vi "Measure.vi"(11 "FFmeter settings":T1={"AC Source"={"AC Source type"=enum."Fluke 5XXX calibrator", "VISA"="", "Ref. clock (Hz)"=0.0, "status ref"=refnum}, "TWM pipe"="\\\\.\\pipe\\TWM:server", "Measurement status ref"=refnum, "TWM Status ref"=refnum, "Abort ref"=refnum, "DC meter"={"DC meter type"=enum."H/A/K 3458", "DC meter VISA"="", "NPLC"=10, "No of readings"=3, "status ref"=refnum}, "Measurement properties"={"Measurement frequencies (Hz)"=[1000.0], "Sampling frequency (Hz)"=500000.0, "Signal amplitude (V)"=4.5, "AC-DC settle time (s)"=20.0, "Record length (multiples of period)"=[1000.0, 10000.0, 1000.0], "Measurement template file"=path "", "Row of START keyword"=1, "Row of STOP keyword"=0, "Calculate RMS from samples"=FALSE}} {"Measurement properties"."Record length (multiples of period)" format="%#_3p"; "Measurement properties"."Sampling frequency (Hz)" format="%#_3p"; "Measurement properties"."Measurement frequencies (Hz)" format="%#_3p"}) -> (0 "error out":errorcluster, 3 "FFmeter settings out":T1={"AC Source"={"AC Source type"=enum."Fluke 5XXX calibrator", "VISA"="", "Ref. clock (Hz)"=0.0, "status ref"=refnum}, "TWM pipe"="\\\\.\\pipe\\TWM:server", "Measurement status ref"=refnum, "TWM Status ref"=refnum, "Abort ref"=refnum, "DC meter"={"DC meter type"=enum."H/A/K 3458", "DC meter VISA"="", "NPLC"=10, "No of readings"=3, "status ref"=refnum}, "Measurement properties"={"Measurement frequencies (Hz)"=[1000.0], "Sampling frequency (Hz)"=500000.0, "Signal amplitude (V)"=4.5, "AC-DC settle time (s)"=20.0, "Record length (multiples of period)"=[1000.0, 10000.0, 1000.0], "Measurement template file"=path "", "Row of START keyword"=1, "Row of STOP keyword"=0, "Calculate RMS from samples"=FALSE}} {"Measurement properties"."Record length (multiples of period)" format="%#_3p"; "Measurement properties"."Sampling frequency (Hz)" format="%#_3p"; "Measurement properties"."Measurement frequencies (Hz)" format="%#_3p"})   [LabVIEW 2020]
uses:
  GUI/Type definitions/FFmeter settings.ctl
  General AC source/Type definitions/AC Source.ctl
  General AC source/Type definitions/AC Source type.ctl
  General DC meter/Type definitions/DC meter.ctl
  General DC meter/Type definitions/DC meter type.ctl
  Type definitions/Measuement properties.ctl
  <vilib>/Utility/error.llb/DialogType.ctl
  <vilib>/Utility/NIReport.llb/NI_report.lvclass
  external libraries/varilib/varilib.lvlib
  external libraries/TWM-1.8.7.0-client/TWM Client.lvlib
panel:
  out "offset after":dbl[](array[numeric])
  out "DC readings of AC-AC sequence":dbl[][](array[numeric])
  out "offset before":dbl[](array[numeric])
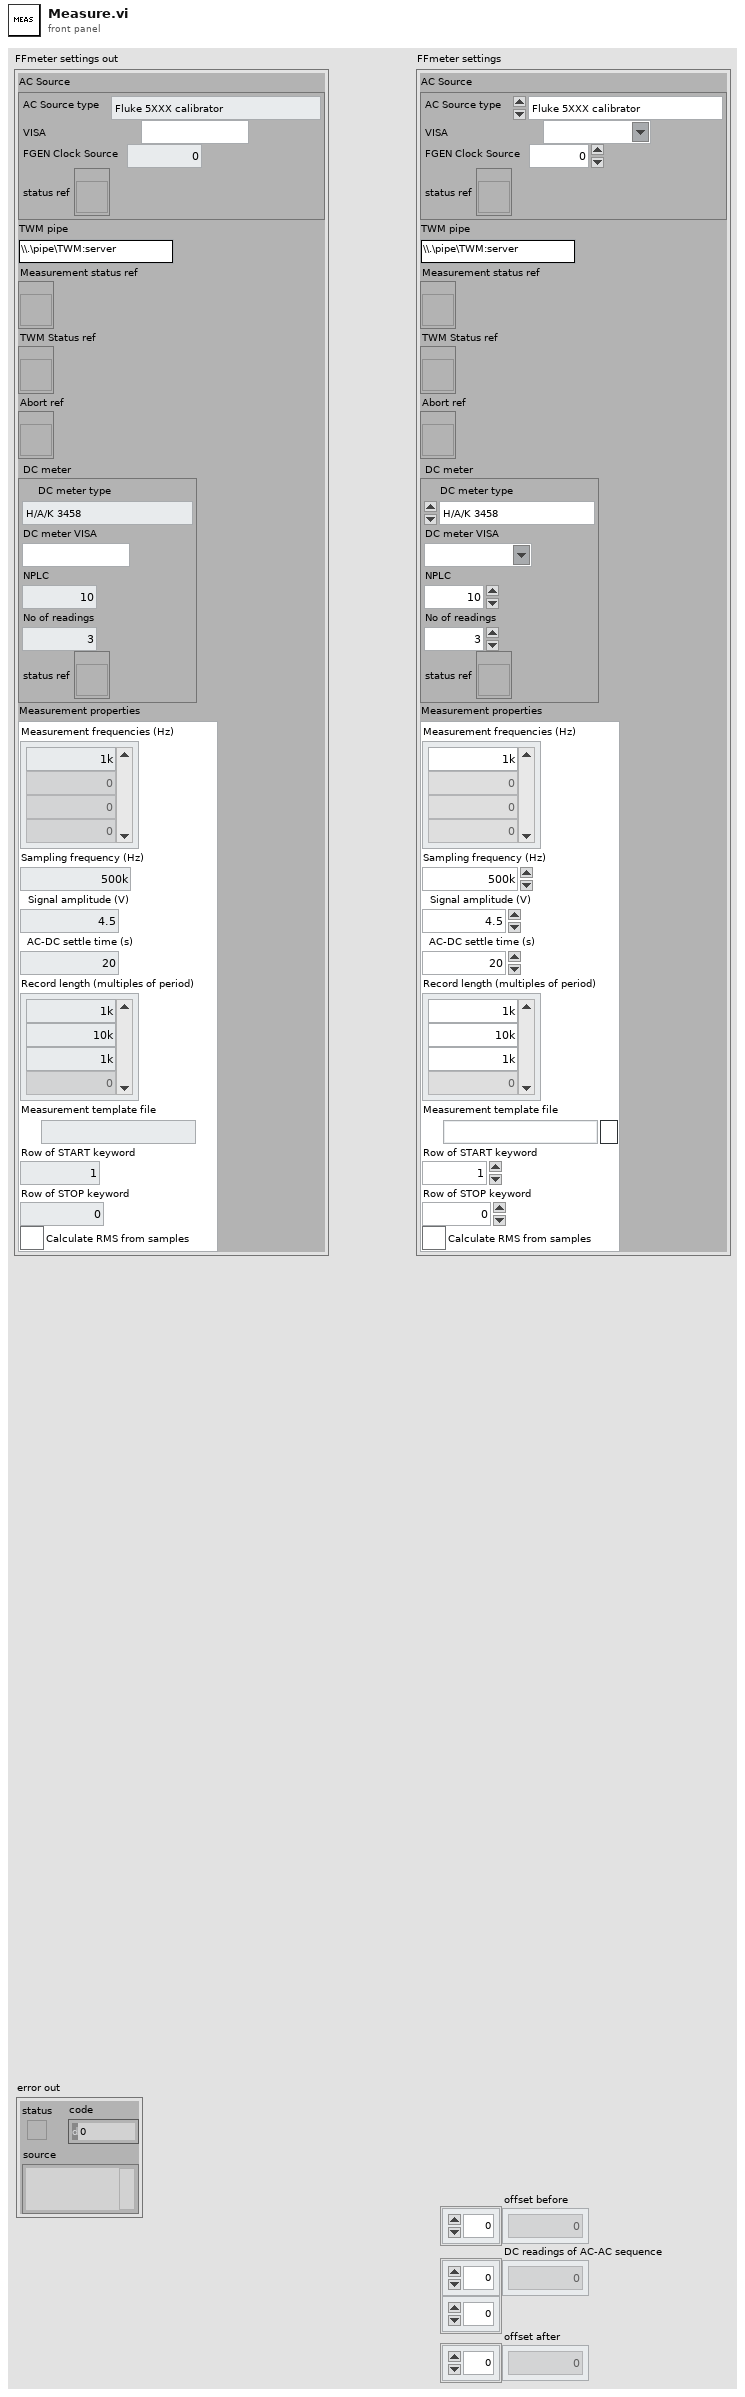
[diagram p1: front panel]
types:
  T1 = typedef "FFmeter settings.ctl" = cluster{"AC Source":T2, "TWM pipe":string, "Measurement status ref":refnum<vi>, "TWM Status ref":refnum<vi>, "Abort ref":refnum<vi>, "DC meter":T4, "Measurement properties":T6}
  T2 = typedef "AC Source.ctl" = cluster{"AC Source type":T3, "VISA":refnum<visa-resource-name>, "Ref. clock (Hz)":dbl, "status ref":refnum<vi>}
  T3 = typedef "AC Source type.ctl" = enum16{"Fluke 5XXX calibrator", "Tektronix AFG3101C", "dummy"}
  T4 = typedef "DC meter.ctl" = cluster{"DC meter type":T5, "DC meter VISA":refnum<visa-resource-name>, "NPLC":i32, "No of readings":i32, "status ref":refnum<vi>}
  T5 = typedef "DC meter type.ctl" = enum16{"H/A/K 3458", "FLuke 8508A", "dummy"}
  T6 = typedef "Measuement properties.ctl" = cluster{"Measurement frequencies (Hz)":dbl[], "Sampling frequency (Hz)":dbl, "Signal amplitude (V)":dbl, "AC-DC settle time (s)":dbl, "Record length (multiples of period)":dbl[], "Measurement template file":path, "Row of START keyword":i32, "Row of STOP keyword":i32, "Calculate RMS from samples":bool}
  T7 = typedef "DialogType.ctl" = u16
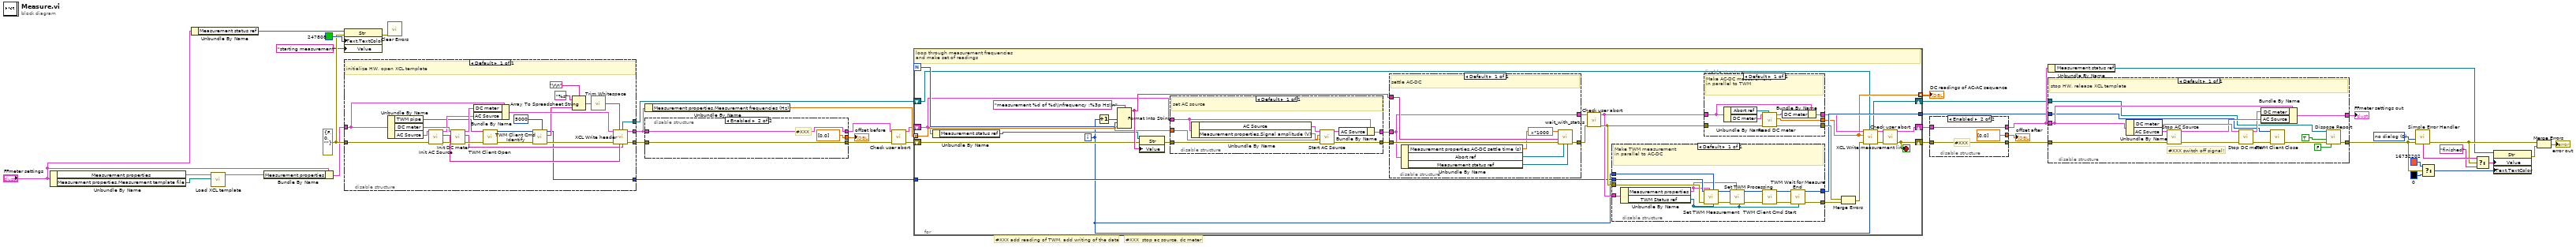
[diagram p0: block diagram]
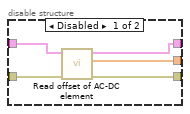
[diagram p2: hidden frame]
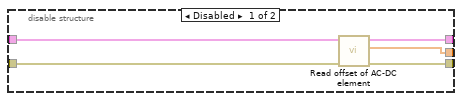
[diagram p3: hidden frame]
diagram:
  w32 = T7 0 items=["no dialog", "OK message", "continue or stop message", "OK message + warnings", "continue/stop + warnings"] ("type of dialog (OK msg:1)")
  w7 = errorcluster {"status"=FALSE, "code"=0, "source"=""} ("error out")
  # "#XXX  stop ac source, dc meter"
  # "#XXX add reading of TWM, add writing of the data"
  n1 = Unbundle By Name("FFmeter settings") -> ("Measurement properties"=w5:T6, "Measurement properties.Measurement template file"=w1:path)
  n2 = Unbundle By Name("FFmeter settings") -> ("Measurement status ref"=w24:refnum<vi>)
  n3 = call "Load XCL template.vi"("Measurement template file"=w1, "Measurement properties"=w5) -> ("Measurement properties out"=w4:T6)  [unwired: 9 in]
  n4 = Bundle By Name(cluster="FFmeter settings", "Measurement properties"=w4) -> (w2:T1)
  n5 = property class="Str"(reference=w24, error in=w7, "Text.TextColor"=u32 247808 ("Text.Text Colors:Text Color"), "Value"="starting measurement") -> (error out=w23:errorcluster)  [unwired: 1 out]
  n6 = disable-structure shown="Default" {
    disable-tunnel: w2 -> [w63]
    disable-tunnel: [w54] -> w9
    disable-tunnel: w7 -> [w60]
    disable-tunnel: [w57] -> w11
    disable-tunnel: [w45] -> w15
    disable-tunnel: [w55] -> w13
    frame Enabled {
      # "initialize HW, open XCL template"
      n7 = Unbundle By Name(w63) -> ("TWM pipe"=w58:string, "DC meter"=w64:T4, "AC Source"=w65:T2)
      n8 = call "Init AC Source.vi"("error in (no error)"=w60, "AC source"=w65) -> ("error out"=w66:errorcluster, "Init status"=w53:string, "AC source out"=w61:T2)  [unwired: 7 in]
      n9 = call "Init DC meter.vi"("error in (no error)"=w66, "DC meter"=w64) -> ("error out"=w59:errorcluster, "Init status"=w52:string, "DC meter out"=w62:T4)  [unwired: 7 in]
      n10 = Bundle By Name(cluster=w63, "DC meter"=w62, "AC Source"=w61) -> (w56:T1)
      n11 = call "TWM Client Open.vi"("error in"=w59, "pipe name"=w58) -> ("error out"=w47:errorcluster, "handle out"=w48:i32)  [unwired: 8 in]
      n12 = call "TWM Client Cmd Identify.vi"("timeout [ms]"=5000, "error in"=w47, "handle"=w48) -> ("error out"=w46:errorcluster, "channel idns"=w51:string[], "handle out"=w45:i32)  [unwired: 5 in, 1 out]
      n13 = Array To Spreadsheet String(delimiter (Tab)="\r\n", array=w51, 3:"%s" ("format string")) -> (spreadsheet string=w44:string)
      n14 = call <vilib>:"Trim Whitespace.vi"("string"=w44) -> ("trimmed string"=w43:string)  [unwired: 1 in]
      n15 = call "XCL Write header.vi"("DC meter idn"=w52, "AC source idn"=w53, "Digitizer idn"=w43, "error in (no error)"=w46, "FFmeter settings"=w56) -> ("error out"=w57:errorcluster, "FFmeter settings out"=w54:T1, "NI_report out"=w55:refnum<class "NI_report.lvclass">)  [unwired: 4 in]
    }
  }
  n16 = call <vilib>:"Clear Errors.vi"("error in (no error)"=w23) -> ()  [unwired: 5 in, 2 out]
  n17 = Unbundle By Name(w9) -> ("Measurement properties.Measurement frequencies (Hz)"=w41:dbl[])
  n18 = disable-structure shown="Enabled" {
    disable-tunnel: [w71 w72] -> w10
    disable-tunnel: w11 -> [w70 w72]
    disable-tunnel: w9 -> [w69 w74]
    disable-tunnel: [w68 dbl[] [0.0] ("offset before")] -> w39
    disable-tunnel: [w67 w74] -> w8
    frame Disabled {
      n19 = call "Read offset of AC-DC element.vi"("error in (no error)"=w70, "FFmeter settings in"=w69) -> ("error out"=w71:errorcluster, "DC readings"=w68:dbl[], "FFmeter settings out"=w67:T1)  [unwired: 7 in]
    }
    frame Enabled {
      # "#XXX"
    }
  }
  "offset before" <- w39
  n20 = call "Check user abort.vi"("error in (no error)"=w10, "FFmeter settings"=w8) -> ("error out"=w22:errorcluster, "FFmeter settings out"=w21:T1)  [unwired: 8 in]
  n21 = for {
    N -> [w100]
    shift-right: [w86] -> w37
    shift-left: w22 -> [w92]
    shift-right: [w85] -> w38
    shift-left: w21 -> [w91]
    tunnel: w41 -> [w93] mode=indexing
    tunnel: [w81] -> w40 mode=indexing
    tunnel: w15 -> [w84]
    tunnel: [w83] -> w14
    shift-right: [w76] -> w12
    shift-left: w13 -> [w75]
    i -> [w77]
    stop <- w86 stop-if-true
    # "loop through measurement frequencies\nand make set of readings"
    n22 = Unbundle By Name(w91) -> ("Measurement status ref"=w97:refnum<vi>)
    n23 = Increment(x=w77) -> (x+1=w101:i32)
    n24 = Format Into String(format string="measurement %d of %d\\nfrequency :%3p Hz\\n", w101, w100, w93) -> (resulting string=w102:string)  [unwired: 2 in, 1 out]
    n25 = property class="Str"(reference=w97, error in=w92, "Value"=w102) -> (error out=w96:errorcluster)  [unwired: 1 out]
    n26 = disable-structure shown="Default" {
      disable-tunnel: w91 -> [w118]
      disable-tunnel: w96 -> [w117]
      disable-tunnel: [w116] -> w95
      disable-tunnel: [w119] -> w94
      disable-tunnel: w93 -> [w113]
      frame Enabled {
        # "set AC source"
        n27 = Unbundle By Name(w118) -> ("AC Source"=w114:T2, "Measurement properties.Signal amplitude (V)"=w112:dbl)
        n28 = call "Start AC Source.vi"("error in (no error)"=w117, "Signal amplitude (V)"=w112, "Signal frequency  (Hz)"=w113, "AC source"=w114) -> ("error out"=w116:errorcluster, "AC source out"=w115:T2)  [unwired: 5 in, 1 out]
        n29 = Bundle By Name(cluster=w118, "AC Source"=w115) -> (w119:T1)
      }
    }
    n30 = disable-structure shown="Default" {
      disable-tunnel: w102 -> [w111]
      disable-tunnel: [w104] -> w90
      disable-tunnel: [w109] -> w87
      disable-tunnel: w95 -> [w110]
      disable-tunnel: w94 -> [w109]
      frame Enabled {
        # "settle AC-DC"
        n31 = Unbundle By Name(w109) -> ("Measurement properties.AC-DC settle time (s)"=w107:dbl, "Abort ref"=w106:refnum<vi>, "Measurement status ref"=w105:refnum<vi>)
        n32 = expression code="x*1000"(w107) -> (w108:dbl)
        n33 = call "wait_with_status.vi"("stat ref"=w105, "stop ref"=w106, "error in"=w110, "comment"=w111, "ms to wait"=w108) -> ("error out"=w104:errorcluster)  [unwired: 5 in, 1 out]
      }
    }
    n34 = call "Check user abort.vi"("error in (no error)"=w90, "FFmeter settings"=w87) -> ("error out"=w89:errorcluster, "FFmeter settings out"=w88:T1)  [unwired: 8 in]
    n35 = disable-structure shown="Default" {
      disable-tunnel: [w136] -> w98
      disable-tunnel: w89 -> [w135]
      disable-tunnel: w88 -> [w141]
      disable-tunnel: w84 -> [w134]
      disable-tunnel: [w137] -> w83
      disable-tunnel: w77 -> [w140]
      frame Enabled {
        # "Make TWM measurement\nin parallel to AC-DC"
        n36 = Unbundle By Name(w141) -> ("Measurement properties"=w129:T6, "TWM Status ref"=w128:refnum<vi>)
        n37 = call "Set TWM Measurement.vi"("status ref (none)"=w128, "Loop iteration"=w140, "Measurement properties"=w129, "error in"=w135, "handle"=w134) -> ("error out"=w133:errorcluster, "handle out"=w130:i32)  [unwired: 5 in]
        n38 = call "Set TWM Processing.vi"("status ref (none)"=w128, "Measurement properties"=w129, "error in"=w133, "handle"=w130) -> ("error out"=w132:errorcluster, "handle out"=w131:i32)  [unwired: 6 in]
        n39 = call "TWM Client Cmd Start.vi"("error in"=w132, "handle"=w131) -> ("error out"=w139:errorcluster, "handle out"=w138:i32)  [unwired: 8 in]
        n40 = call "TWM Wait for Measure End.vi"("handle"=w138, "error in"=w139, "status ref (none)"=w128) -> ("handle out"=w137:i32, "error out"=w136:errorcluster)  [unwired: 8 in, 3 out]
      }
    }
    n41 = disable-structure shown="Default" {
      disable-tunnel: [w127] -> w81
      disable-tunnel: [w126] -> w99
      disable-tunnel: w89 -> [w125]
      disable-tunnel: w88 -> [w122]
      disable-tunnel: [w121] -> w82
      frame Enabled {
        # "Make AC-DC measurement\nin parallel to TWM"
        n42 = Unbundle By Name(w122) -> ("Abort ref"=w120:refnum<vi>, "DC meter"=w124:T4)
        n43 = call "Read DC meter.vi"("abort reference"=w120, "error in (no error)"=w125, "DC meter"=w124) -> ("error out"=w126:errorcluster, "DC readings"=w127:dbl[], "DC meter out"=w123:T4)  [unwired: 6 in]
        n44 = Bundle By Name(cluster=w122, "DC meter"=w123) -> (w121:T1)
      }
    }
    n45 = Merge Errors(w99, w98) -> (w80:errorcluster)
    n46 = call "XCL Write measurement line.vi"("Iteration index"=w77, "report in"=w75, "error in (no error)"=w80, "DC readings"=w81, "FFmeter settings in"=w82) -> ("error out"=w79:errorcluster, "FFmeter settings out"=w78:T1, "report out"=w76:refnum<class "NI_report.lvclass">)  [unwired: 4 in]
    n47 = call "Check user abort.vi"("error in (no error)"=w79, "FFmeter settings"=w78) -> ("error out"=w86:errorcluster, "FFmeter settings out"=w85:T1)  [unwired: 8 in]
  }
  "DC readings of AC-AC sequence" <- w40
  n48 = disable-structure shown="Enabled" {
    disable-tunnel: w38 -> [w146 w149]
    disable-tunnel: [w145 w149] -> w17
    disable-tunnel: w37 -> [w144 w147]
    disable-tunnel: [w143 w147] -> w19
    disable-tunnel: [w142 dbl[] [0.0] ("offset after")] -> w36
    frame Disabled {
      n49 = call "Read offset of AC-DC element.vi"("error in (no error)"=w144, "FFmeter settings in"=w146) -> ("error out"=w143:errorcluster, "DC readings"=w142:dbl[], "FFmeter settings out"=w145:T1)  [unwired: 7 in]
    }
    frame Enabled {
      # "#XXX"
    }
  }
  "offset after" <- w36
  n50 = Unbundle By Name(w17) -> ("Measurement status ref"=w20:refnum<vi>)
  n51 = disable-structure shown="Default" {
    disable-tunnel: w17 -> [w164]
    disable-tunnel: [w163] -> w16
    disable-tunnel: [w153] -> w18
    disable-tunnel: w19 -> [w157]
    disable-tunnel: w14 -> [w155]
    disable-tunnel: w12 -> [w152]
    frame Enabled {
      # "#XXX switch off signal!"
      # "stop HW, release XCL template"
      n52 = Unbundle By Name(w164) -> ("DC meter"=w160:T4, "AC Source"=w161:T2)
      n53 = call "Stop AC Source.vi"("error in (no error)"=w157, "AC source"=w161) -> ("error out"=w162:errorcluster, "AC source out"=w159:T2)  [unwired: 8 in]
      n54 = call "Stop DC meter.vi"("error in (no error)"=w162, "DC meter"=w160) -> ("error out"=w156:errorcluster, "DC meter out"=w158:T4)  [unwired: 8 in]
      n55 = Bundle By Name(cluster=w164, "DC meter"=w158, "AC Source"=w159) -> (w163:T1)
      n56 = call "TWM Client Close.vi"("error in"=w156, "handle in"=w155) -> ("error out"=w154:errorcluster)  [unwired: 9 in]
      n57 = call-dynamic "Dispose Report.vi"("report in"=w152, "save changes? (F)"=TRUE, "error in (no error)"=w154, "close report? (T)"=FALSE) -> ("error out"=w153:errorcluster)  [unwired: 11 in]
    }
  }
  "FFmeter settings out" <- w16
  n58 = call <vilib>:"Simple Error Handler.vi"("type of dialog (OK msg:1)"=w32, "error in (no error)"=w18) -> ("error out"=w27:errorcluster, "message"=w35:string)  [unwired: 3 in, 3 out]
  n59 = Select(t=u32 16732202 ("Text.Text Colors:Text Color"), s=w18, f=u32 0 ("Text.Text Colors:Text Color")) -> (s? t:f=w29:u32)
  n60 = Select(t=w35, s=w27, f="finished") -> (s? t:f=w33:string)
  n61 = property class="Str"(reference=w20, "Value"=w33, "Text.TextColor"=w29) -> (error out=w28:errorcluster)  [unwired: 1 in, 1 out]
  n62 = Merge Errors(w27, w28) -> (→"error out":errorcluster)
